vi "ex_1_ES_main.vi"() -> ()   [LabVIEW 2020]
uses:
  #typedef_Sound_Intensity.ctl
  <vilib>/Utility/miscctls.llb/LVPositionTypeDef.ctl
  ex_2/#typedef_ProgramData.ctl
panel:
  in  "Position":T1
  out "To be moved":string
  in  "Sound intensity: MAX":dbl=100.0
  in  "Sound intensity: MIN":dbl
  out "Limit exceeded?":bool
  in  "Stop Button":bool
  in  "Sound intensity [dB]":T2 scale=0.0..100.0
  # "85 dB"
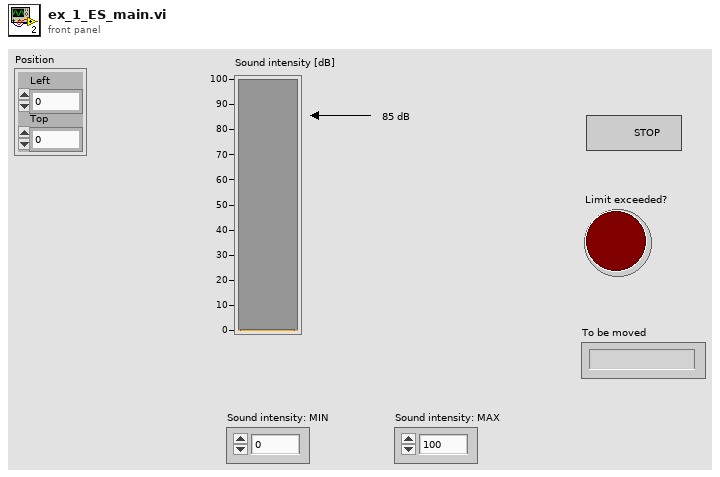
[diagram p1: front panel]
types:
  T1 = typedef "LVPositionTypeDef.ctl" = cluster{"Left":i32, "Top":i32}
  T2 = typedef "#typedef_Sound_Intensity.ctl" = dbl
  T3 = typedef "#typedef_ProgramData.ctl" = cluster{"MousePressed?":bool, "Keyboard":string}
  T4 = typedef "LVPoint32TypeDef.ctl" = cluster{"Horizontal":i32, "Vertical":i32}
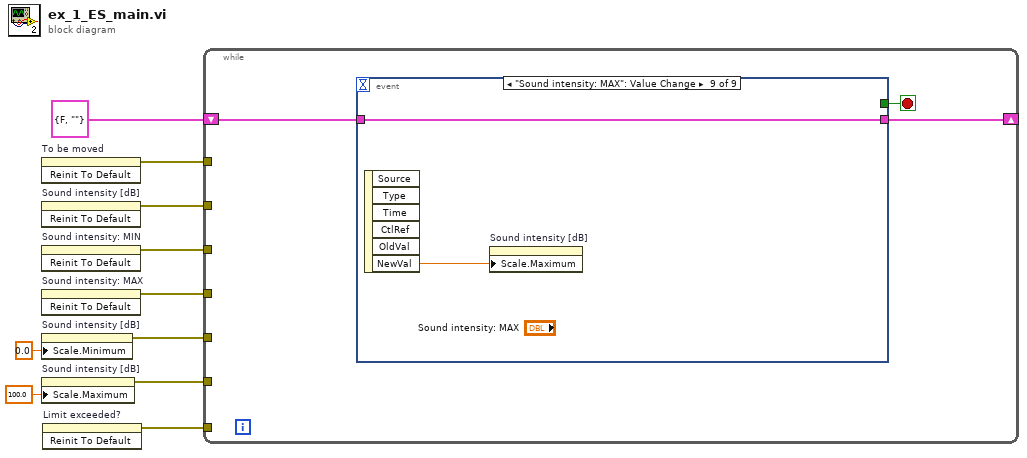
[diagram p0: block diagram]
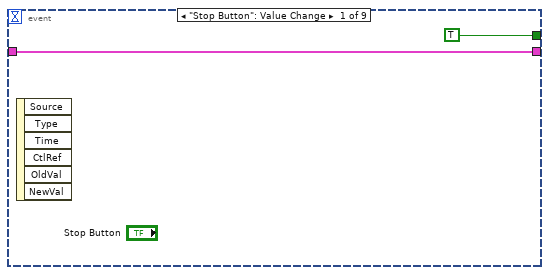
[diagram p2: hidden frame]
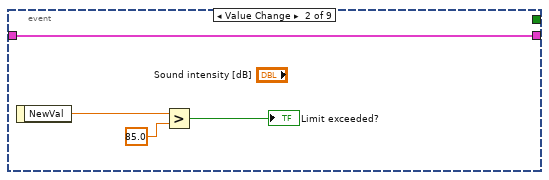
[diagram p3: hidden frame]
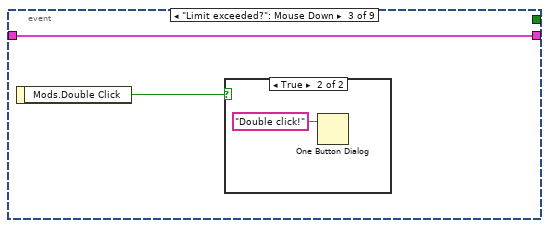
[diagram p4: hidden frame]
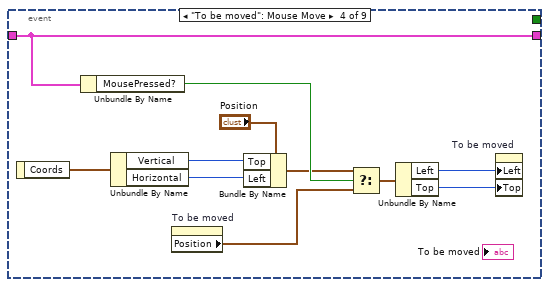
[diagram p6: hidden frame]
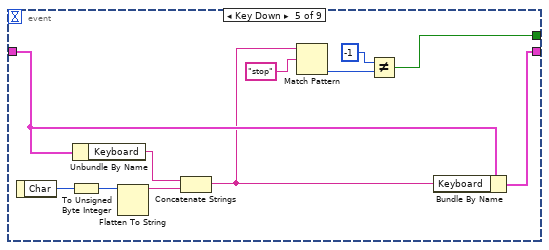
[diagram p7: hidden frame]
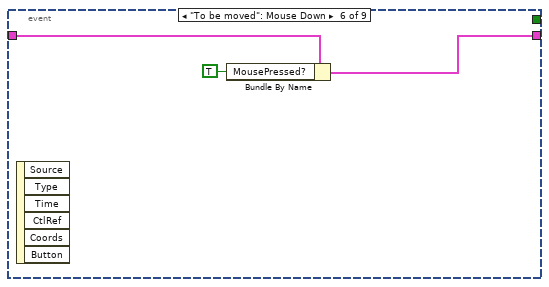
[diagram p8: hidden frame]
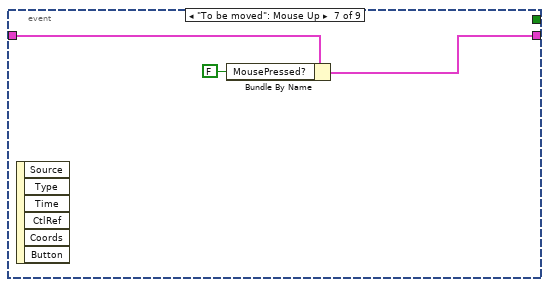
[diagram p9: hidden frame]
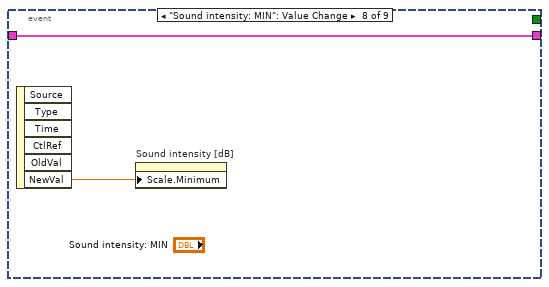
[diagram p10: hidden frame]
diagram:
  n1 = invoke on="To be moved" class="Str" method="Reinit To Default"() -> (error out=w9:errorcluster)  [unwired: 3 in, 2 out]
  n2 = invoke on="Sound intensity [dB]" class="Slide (strict)" method="Reinit To Default"() -> (error out=w8:errorcluster)  [unwired: 3 in, 2 out]
  n3 = invoke on="Sound intensity: MIN" class="DigNum (strict)" method="Reinit To Default"() -> (error out=w7:errorcluster)  [unwired: 3 in, 2 out]
  n4 = invoke on="Sound intensity: MAX" class="DigNum (strict)" method="Reinit To Default"() -> (error out=w6:errorcluster)  [unwired: 3 in, 2 out]
  n5 = property on="Sound intensity [dB]" class="Slide (strict)"("Scale.Minimum"=0.0 ("Scale.Range:Minimum")) -> (error out=w5:errorcluster)  [unwired: 2 in, 1 out]
  n6 = property on="Sound intensity [dB]" class="Slide (strict)"("Scale.Maximum"=100.0 ("Scale.Range:Maximum")) -> (error out=w4:errorcluster)  [unwired: 2 in, 1 out]
  n7 = invoke on="Limit exceeded?" class="Bool (strict)" method="Reinit To Default"() -> (error out=w1:errorcluster)  [unwired: 3 in, 2 out]
  n8 = while {
    shift-right: [w11] -> _
    shift-left: T3 {"MousePressed?"=FALSE, "Keyboard"=""} ("ProgramData") -> [w12]
    tunnel: w9 -> [_]
    tunnel: w8 -> [_]
    tunnel: w7 -> [_]
    tunnel: w6 -> [_]
    tunnel: w5 -> [_]
    tunnel: w4 -> [_]
    tunnel: w1 -> [_]
    stop <- w13 stop-if-true
    n9 = event shown="[8] \"Sound intensity: MAX\": Value Change" {
      selector: _ -> [_ _ _ _ _ _ _ _ _]
      dyn-events: _ -> [_ _ _ _ _ _ _ _ _]
      timeout: _ -> [_ _ _ _ _ _ _ _ _]
      tunnel: [TRUE _ _ _ w34 _ _ _ _] -> w13
      tunnel: [w14 w16 w20 w31 w39 w46 w49 w51 w53] -> w11
      tunnel: w12 -> [w14 w16 w20 w31 w43 w47 w50 w51 w53]
      event "Stop Button": Value Change {
        n10 = event-data() -> ()  [unwired: 1 in, 6 out]
      }
      event Value Change {
        n11 = event-data() -> ("NewVal"=w19:T2)  [unwired: 1 in]
        n12 = Greater?(x=w19, y=85.0) -> (0:→"Limit exceeded?":bool)
      }
      event "Limit exceeded?": Mouse Down {
        n13 = event-data() -> ("Mods.Double Click"=w21:bool)  [unwired: 1 in]
        n14 = case shown="True" w21 {
          frame False {
          }
          frame True {
            n15 = One Button Dialog(message="Double click!") -> ()  [unwired: 1 in, 1 out]
          }
        }
      }
      event "To be moved": Mouse Move {
        n16 = event-data() -> ("Coords"=w27:T4)  [unwired: 1 in]
        n17 = Unbundle By Name(w31) -> ("MousePressed?"=w29:bool)
        n18 = Unbundle By Name(w27) -> ("Vertical"=w25:i32, "Horizontal"=w24:i32)
        n19 = property on="To be moved" class="Str"() -> ("Position"=w28:T1)  [unwired: 2 in, 2 out]
        n20 = Bundle By Name(cluster="Position", "Top"=w25, "Left"=w24) -> (w23:T1)
        n21 = Select(t=w23, s=w29, f=w28) -> (s? t:f=w30:T1)
        n22 = Unbundle By Name(w30) -> ("Left"=w33:i32, "Top"=w32:i32)
        n23 = property on="To be moved" class="Str"("Left"=w33, "Top"=w32) -> ()  [unwired: 2 in, 2 out]
      }
      event Key Down {
        n24 = event-data() -> ("Char"=w44:i16)  [unwired: 1 in]
        n25 = To Unsigned Byte Integer(number=w44) -> (unsigned 8bit integer=w40:u8)
        n26 = Unbundle By Name(w43) -> ("Keyboard"=w42:string)
        n27 = Flatten To String(anything=w40) -> (data string=w41:string)  [unwired: 3 in, 2 out]
        n28 = Concatenate Strings(w42, w41) -> (w38:string)
        n29 = Match Pattern(string=w38, regular expression="stop") -> (offset past match=w36:i32)  [unwired: 1 in, 3 out]
        n30 = Not Equal?(x=-1, y=w36) -> (x != y?=w34:bool)
        n31 = Bundle By Name(cluster=w43, "Keyboard"=w38) -> (w39:T3)
      }
      event "To be moved": Mouse Down {
        n32 = event-data() -> ()  [unwired: 1 in, 6 out]
        n33 = Bundle By Name(cluster=w47, "MousePressed?"=TRUE) -> (w46:T3)
      }
      event "To be moved": Mouse Up {
        n34 = event-data() -> ()  [unwired: 1 in, 6 out]
        n35 = Bundle By Name(cluster=w50, "MousePressed?"=FALSE) -> (w49:T3)
      }
      event "Sound intensity: MIN": Value Change {
        n36 = event-data() -> ("NewVal"=w52:dbl)  [unwired: 1 in, 5 out]
        n37 = property on="Sound intensity [dB]" class="Slide (strict)"("Scale.Minimum"=w52) -> ()  [unwired: 2 in, 2 out]
      }
      event "Sound intensity: MAX": Value Change {
        n38 = event-data() -> ("NewVal"=w54:dbl)  [unwired: 1 in, 5 out]
        n39 = property on="Sound intensity [dB]" class="Slide (strict)"("Scale.Maximum"=w54) -> ()  [unwired: 2 in, 2 out]
      }
    }
  }
